vi "Download_Manager.vi"(7 "Downloader Exit":refnum<user-event>, 11 "manager_daemon":refnum<class "manager_daemon.lvclass">) -> ()   [LabVIEW 2024, in "Download_Manager.lvlib"]
uses:
  Download_Manager.lvlib
  comic_manager/manager_daemon/manager_daemon.lvclass
  typedefs/job--cluster.ctl
  typedefs/job_type--enum.ctl
  <vilib>/addons/_JKI.lib/REST Client/classes/REST Client/REST Client.lvclass
  comic_manager/manager_daemon/manager_daemon.lvclass/manager_daemon.ctl
  <vilib>/addons/_JKI Toolkits/State Machine/_JKI_lib_State_Machine.llb/Select State(s)_err__jki_lib_state_machine.vi
  <vilib>/Utility/error.llb/Trim Whitespace One-Sided.vi
  CV_RESTful_Library/CV_RESTful_Lib.lvlib
  <userlib>/_OpenG.lib/string/string.llb/openg_string.lvlib
  CV_Shared_Library/CV_Shared_Library.lvlib
panel:
  in  "queue publisher":bool
  in  "Publisher ID":i32=31
  in  "pause":bool
  in  "Volume URL":string
  in  "paste from clipboard":bool
  out "current queue size":i32
  out "Approx Completion":timestamp format="%<%x %X>T"
  out "Crawler Running":bool
  out "Timer":dbl
  in  "add url":bool
  in  "Rebuild Job List":bool=TRUE
  out "files updated":string[](array[string])
  in  "start crawler":bool
  out "status":string
  in  "Exit":bool
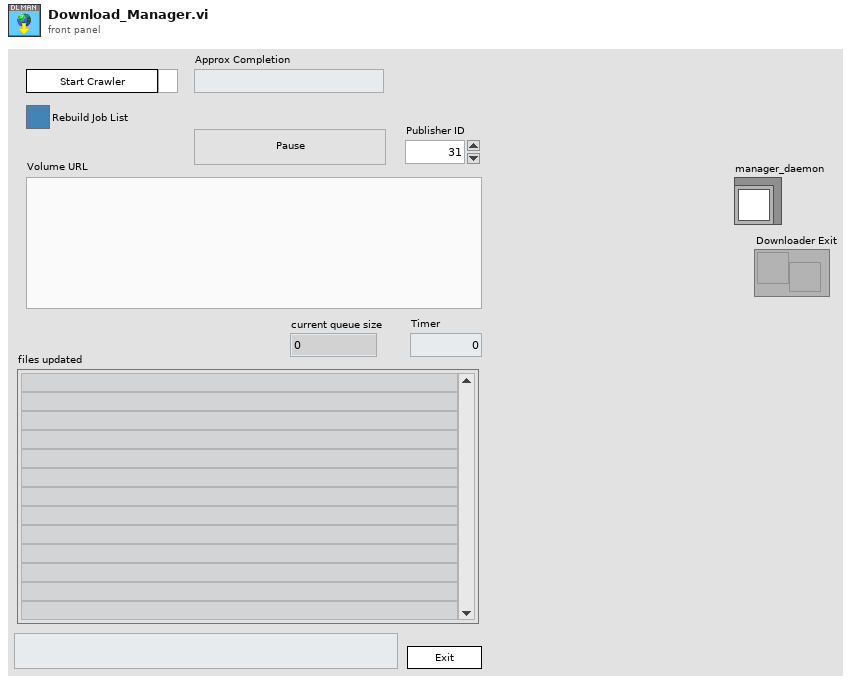
[diagram p1: front panel]
types:
  T1 = typedef "Download_Manager.lvlib/job_type--enum.ctl" = enum16{"check volume date", "check issues date", "download publisher", "download volume", "download isssue"}
  T2 = typedef "Download_Manager.lvlib/job--cluster.ctl" = cluster{"job type":T1, "job path":path, "id":i32, "url":string, "last updated":timestamp, "offset":i32, "original path":path}
  T3 = enum32{"Invalid", "Standard", "Closed", "Hidden", "Minimized", "Maximized"}
  T4 = enum32{"invalid app kind", "Development System", "Run Time System", "Student Edition", "Embedded LabVIEW", "Evaluation", "Custom"}
  T5 = cluster{"Core":cluster{"Current VI Reference":refnum<vi>, "Close Panel on Exit?":bool}, "TO":i32, "dl timer":u32, "cv_vol path":path, "cv_iss path":path, "cache folder":path, "REST Client":refnum<class "REST Client.lvclass">, "crawler active":bool, "job queue":refnum<queue>, "manager_daemon":refnum<class "manager_daemon.lvclass">, "status log ref":refnum<file>, "error log ref":refnum<file>, "ms delay":u32, "cv_pub path":path, "Downloader Exit":refnum<user-event>}
  T6 = cluster{"Current VI Reference":refnum<vi>, "Close Panel on Exit?":bool}
  T7 = typedef "CV_RESTful_Lib.lvlib/local_publisher--cluster.ctl" = cluster{"id":i32, "name":string, "sortable_name":string, "aliases":string[], "description":string, "deck":string, "site_detail_url":string, "date_last_updated":timestamp, "cv_id":string, "volume_ids":i32[]}
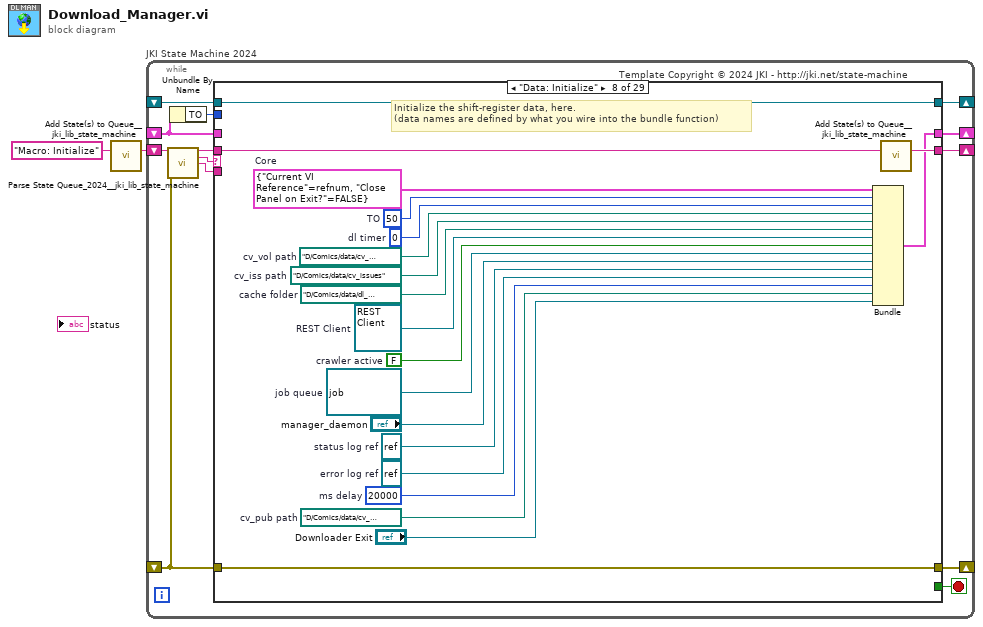
[diagram p0: block diagram]
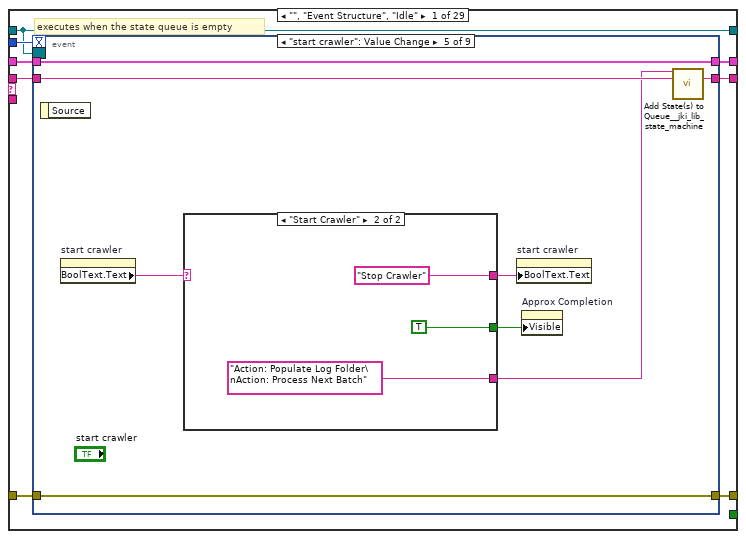
[diagram p2: hidden frame]
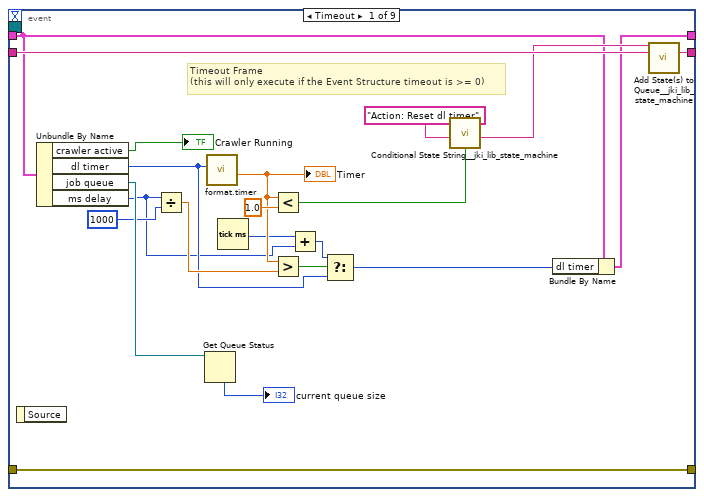
[diagram p3: hidden frame]
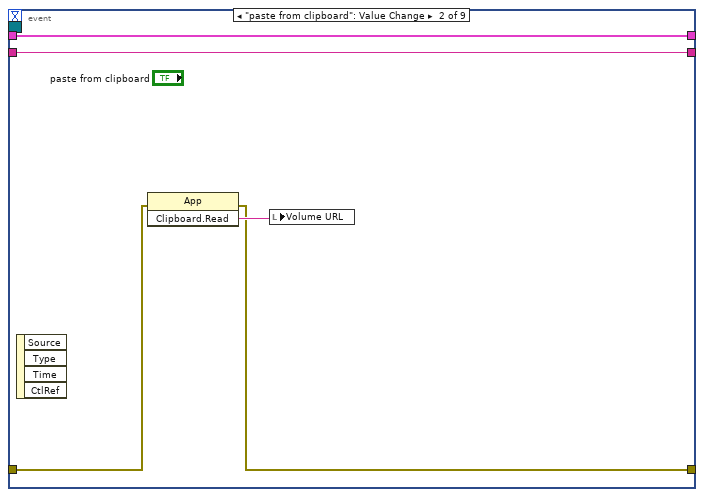
[diagram p4: hidden frame]
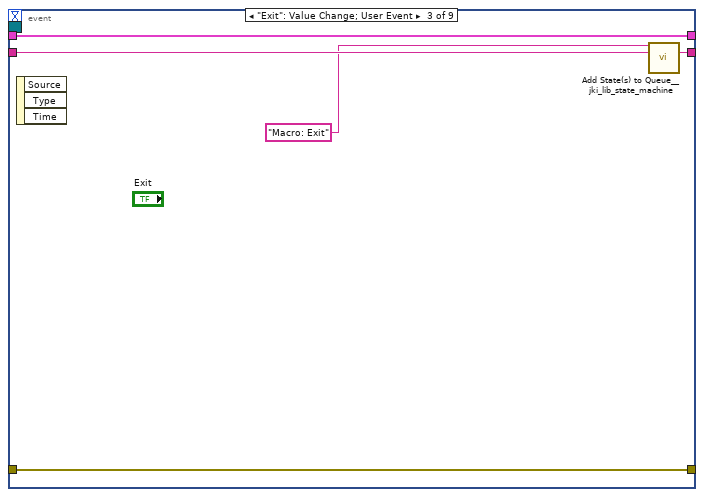
[diagram p5: hidden frame]
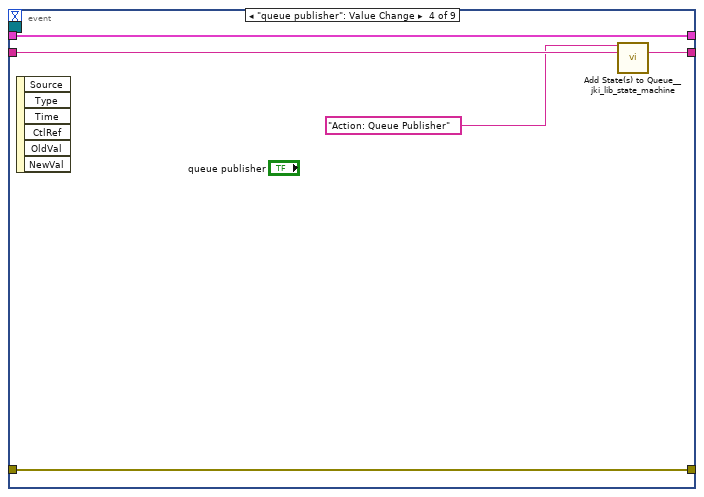
[diagram p6: hidden frame]
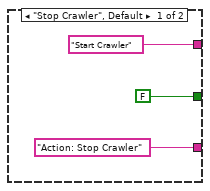
[diagram p7: hidden frame]
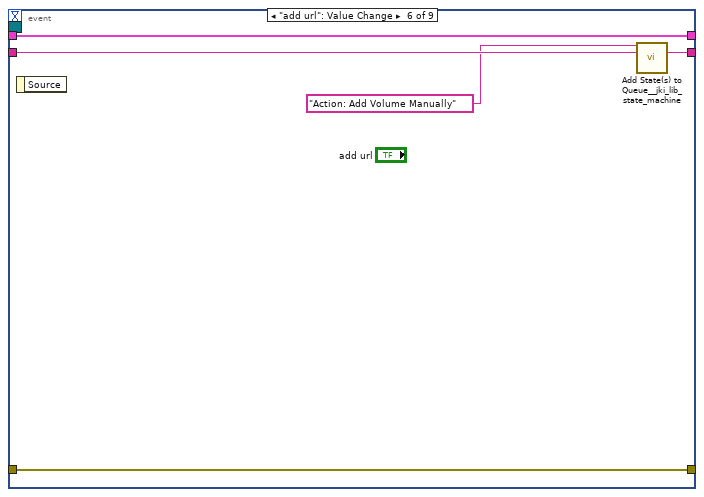
[diagram p8: hidden frame]
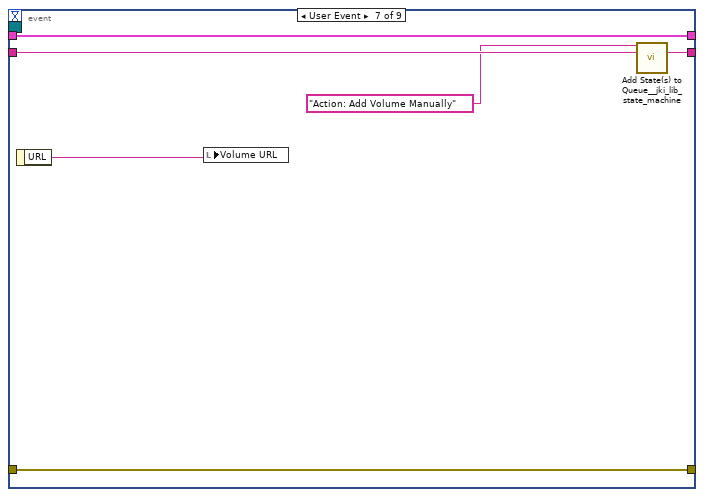
[diagram p9: hidden frame]
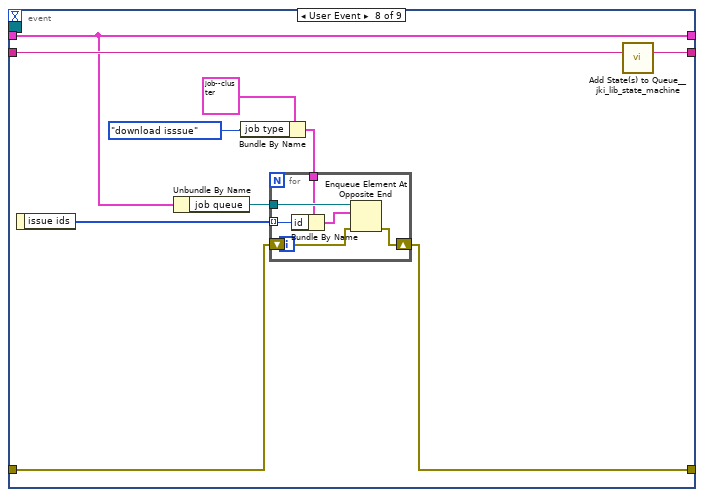
[diagram p10: hidden frame]
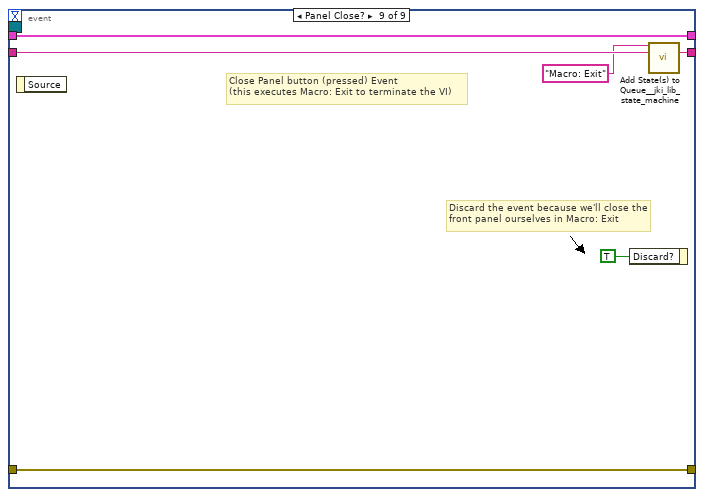
[diagram p11: hidden frame]
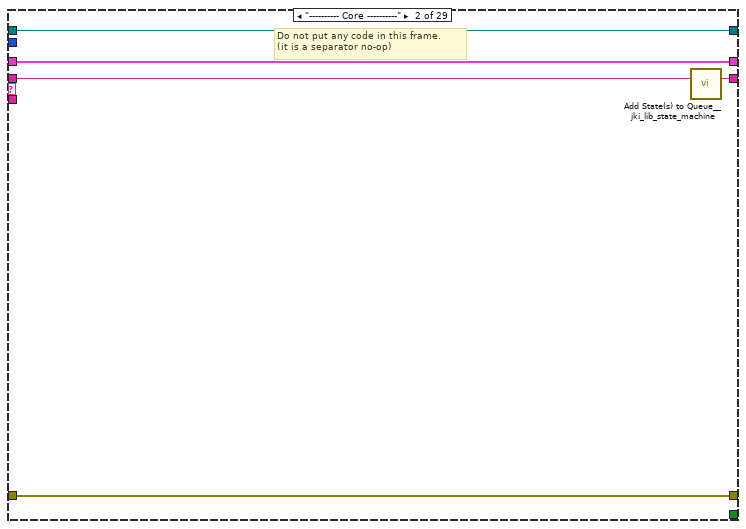
[diagram p12: hidden frame]
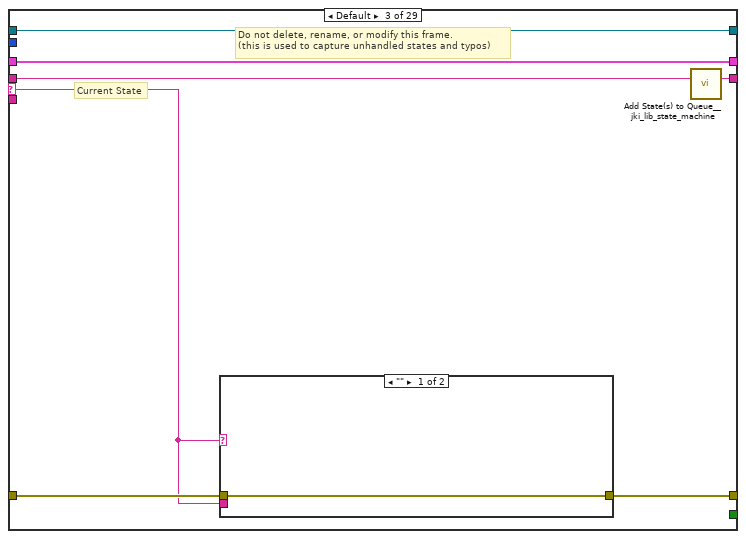
[diagram p13: hidden frame]
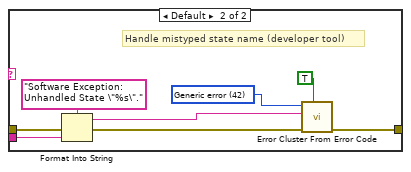
[diagram p14: hidden frame]
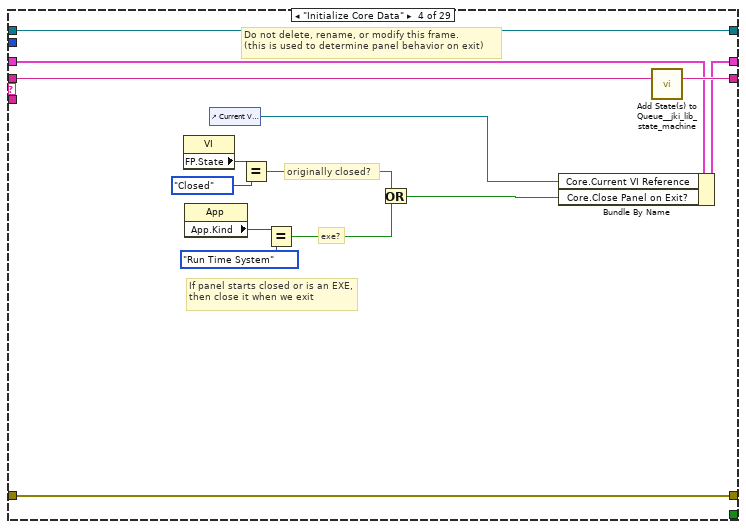
[diagram p15: hidden frame]
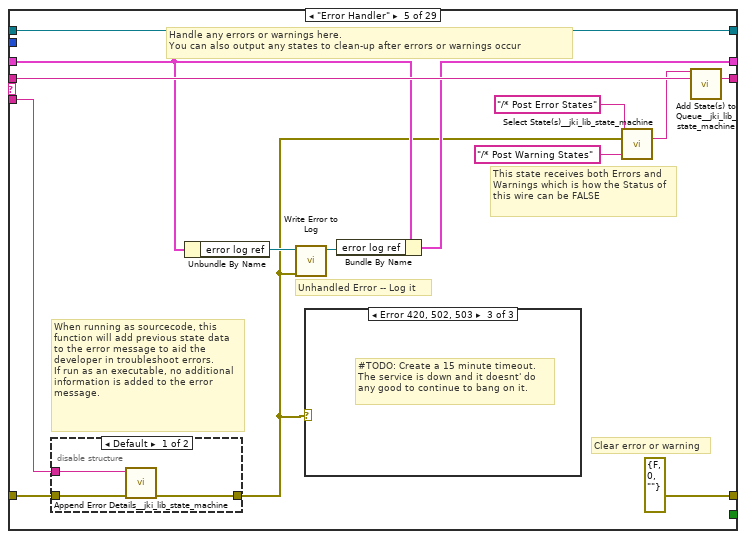
[diagram p16: hidden frame]
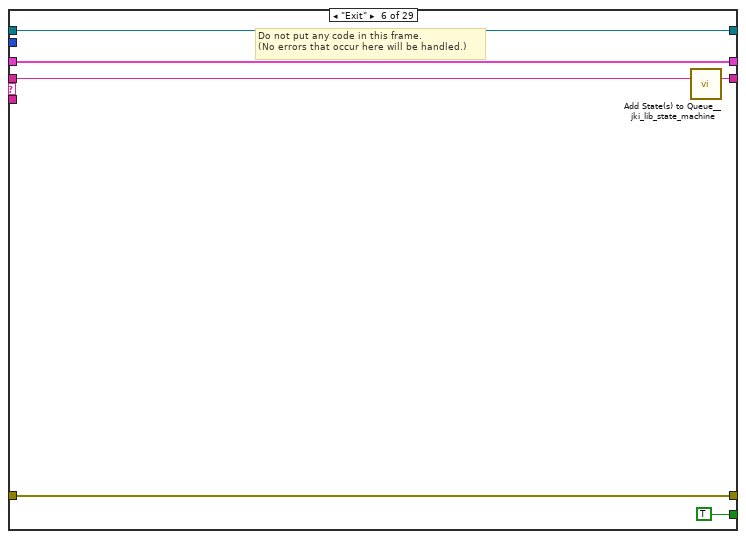
[diagram p20: hidden frame]
diagram:
  n1 = call <vilib>:"Add State(s) to Queue__jki_lib_state_machine.vi"("State(s) in (\"\")"="Macro: Initialize") -> ("States Out"=w2:string)  [unwired: 14 in]
  n2 = while "JKI State Machine 2024" {
    shift-right: [w8] -> _
    shift-left: _ -> [w5]
    shift-right: [w11] -> _
    shift-left: _ -> [w7]
    shift-right: [w10] -> _
    shift-left: w2 -> [w12]
    shift-right: [w4] -> _
    shift-left: _ -> [w3]
    stop <- w9 stop-if-true
    # "Template Copyright © 2024 JKI - http://jki.net/state-machine"
    n3 = call <vilib>:"Parse State Queue_2024__jki_lib_state_machine.vi"("State Queue"=w12, "Error In (no error)"=w7) -> ("Remaining States"=w14:string, "Current State"=w15:string, "Arguments"=w13:string)  [unwired: 11 in]
    n4 = Unbundle By Name(w5) -> ("TO"=w6:i32)
    n5 = case shown="\"Data: Initialize\"" w15 {
      selector: w15 -> [_ _ w113 _ _ _ _ _ _ _ _ _ _ _ _ _ _ _ _ _ _ _ _ _ _ _ _ _ _]
      tunnel: w14 -> [w23 w111 w116 w141 w155 w165 w170 w190 w202 w222 w227 w237 w243 w248 w257 w264 w271 w283 w353 w359 w369 w374 w394 w435 w464 w481 w499 w532 w548]
      tunnel: w13 -> [_ _ _ _ w151 _ _ _ _ _ _ _ _ _ _ _ w266 w277 _ _ _ _ _ _ _ _ _ _ _]
      tunnel: w5 -> [w21 w108 w114 w134 w144 w163 w167 _ w200 w218 w224 w233 w241 w245 w255 w262 w269 w279 w350 w356 w367 w371 w391 w431 w457 w474 w492 w528 w537]
      tunnel: [w20 w109 w118 w138 errorcluster {"status"=FALSE, "code"=0, "source"=""} ("error out") w162 w168 w187 w192 w219 w225 w234 w238 w246 w254 w261 w267 w280 w351 w357 w364 w372 w375 w421 w458 w476 w494 w516 w539] -> w11
      tunnel: w7 -> [w17 w109 w117 w138 w152 w162 w168 w187 w195 w206 w225 w235 w239 w246 w254 w261 w268 w281 w351 w357 w364 w372 w385 w416 w460 w478 w495 w530 w543]
      tunnel: [w22 w110 w115 w140 w154 w164 w169 w189 w201 w221 w226 w236 w242 w247 w256 w263 w270 w282 w352 w358 w368 w373 w393 w434 w463 w480 w498 w531 w547] -> w10
      tunnel: [_ _ _ _ _ TRUE _ _ _ _ _ _ _ _ _ _ _ _ _ _ _ _ _ _ _ _ _ _ _] -> w9
      tunnel: [w19 w108 w114 w139 w145 w163 w167 w188 w199 w218 w224 w233 w241 w245 w255 w262 w269 w279 w350 w356 w367 w371 w391 w424 w457 w474 w493 w527 w536] -> w8
      tunnel: w6 -> [w18 _ _ _ _ _ _ _ _ _ _ _ _ _ _ _ _ _ _ _ _ _ _ _ _ _ _ _ _]
      tunnel: [w16 w107 w112 w128 w143 w160 w166 w173 w191 w209 w223 w228 w240 w244 w250 w258 w265 w276 w349 w354 w360 w370 w392 w418 w456 w471 w490 w511 w533] -> w4
      tunnel: w3 -> [w16 w107 w112 w128 w143 w160 w166 w173 w191 w209 w223 _ w240 w244 w250 w258 w265 w276 w349 w354 w360 w370 w392 w418 w456 w471 w490 w511 w533]
      frame "", "Event Structure", "Idle" {
        # "executes when the state queue is empty"
        n6 = event shown="[4] \"start crawler\": Value Change" {
          selector: w16 -> [_ _ _ _ _ _ _ _ _]
          dyn-events: _ -> [_ _ _ _ _ _ _ _ _]
          timeout: w18 -> [_ _ _ _ _ _ _ _ _]
          tunnel: w23 -> [w44 w48 w54 w58 w67 w77 w83 w94 w106]
          tunnel: [w43 w48 w53 w57 w66 w76 w82 w93 w105] -> w22
          tunnel: w21 -> [w26 w49 w51 w59 w60 w78 w84 w92 w103]
          tunnel: [w42 w46 w52 w55 w65 w74 w80 w85 w104] -> w20
          tunnel: w17 -> [w42 w45 w52 w55 w65 w74 w80 w86 w104]
          tunnel: [w24 w49 w51 w59 w60 w78 w84 w92 w103] -> w19
          event Timeout {
            # "Timeout Frame\n(this will only execute if the Event Structure timeout is >= 0)"
            n7 = event-data() -> ()  [unwired: 1 in, 1 out]
            n8 = Unbundle By Name(w26) -> ("crawler active"=→"Crawler Running":bool, "dl timer"=w30:u32, "job queue"=w36:refnum<queue>, "ms delay"=w28:u32)
            n9 = Divide(x=w28, y=u32 1000) -> (x/y=w32:dbl)
            n10 = Get Queue Status(queue=w36) -> (# elements in queue=→"current queue size":i32)  [unwired: 2 in, 7 out]
            n11 = call "format.timer.vi"("dl timer"=w30) -> ("seconds"=w34:dbl)  [unwired: 10 in]
            "Timer" <- w34
            n12 = Tick Count (ms)() -> (millisecond timer value=w29:u32)
            n13 = Less?(x=w34, y=1.0) -> (x < y?=w40:bool)
            n14 = Greater?(x=w34, y=w32) -> (0:w31:bool)
            n15 = Add(x=w29, y=w28) -> (x+y=w27:u32)
            n16 = Select(t=w27, s=w31, f=w30) -> (s? t:f=w25:u32)
            n17 = call <vilib>:"Conditional State String__jki_lib_state_machine.vi"("Do State(s)?"=w40, "State"="Action: Reset dl timer") -> ("State Out"=w39:string)  [unwired: 7 in]
            n18 = Bundle By Name(cluster=w26, "dl timer"=w25) -> (w24:T5)
            n19 = call <vilib>:"Add State(s) to Queue__jki_lib_state_machine.vi"("State(s) in Front (\"\")"=w39, "State(s) in (\"\")"=w44) -> ("States Out"=w43:string)  [unwired: 13 in]
          }
          event "paste from clipboard": Value Change {
            n20 = event-data() -> ()  [unwired: 1 in, 4 out]
            n21 = invoke class="App" method="Clipboard.Read"(error in=w45) -> (error out=w46:errorcluster, "Read Clipbrd"=w47:string)  [unwired: 2 in, 1 out]
            n22 = local write "Volume URL"(w47) -> ()
          }
          event "Exit": Value Change; User Event {
            n23 = event-data() -> ()  [unwired: 1 in, 3 out]
            n24 = call <vilib>:"Add State(s) to Queue__jki_lib_state_machine.vi"("State(s) in Front (\"\")"="Macro: Exit", "State(s) in (\"\")"=w54) -> ("States Out"=w53:string)  [unwired: 13 in]
          }
          event "queue publisher": Value Change {
            n25 = event-data() -> ()  [unwired: 1 in, 6 out]
            n26 = call <vilib>:"Add State(s) to Queue__jki_lib_state_machine.vi"("State(s) in Front (\"\")"="Action: Queue Publisher" ("State(s) in Front (\"\")"), "State(s) in (\"\")"=w58) -> ("States Out"=w57:string)  [unwired: 13 in]
          }
          event "start crawler": Value Change {
            n27 = event-data() -> ()  [unwired: 1 in, 1 out]
            n28 = property on="start crawler" class="Bool"() -> ("BoolText.Text"=w63:string)  [unwired: 2 in, 2 out]
            n29 = case shown="\"Start Crawler\"" w63 {
              tunnel: ["Action: Stop Crawler" "Action: Populate Log Folder\nAction: Process Next Batch"] -> w64
              tunnel: [FALSE ("Visible") TRUE ("Visible")] -> w62
              tunnel: ["Start Crawler" ("Boolean Text.Text") "Stop Crawler" ("Boolean Text.Text")] -> w61
              frame "Stop Crawler", Default {
              }
              frame "Start Crawler" {
              }
            }
            n30 = property on="start crawler" class="Bool"("BoolText.Text"=w61) -> ()  [unwired: 2 in, 2 out]
            n31 = property on="Approx Completion" class="AbsTime (strict)"("Visible"=w62) -> ()  [unwired: 2 in, 2 out]
            n32 = call <vilib>:"Add State(s) to Queue__jki_lib_state_machine.vi"("State(s) in Front (\"\")"=w64, "State(s) in (\"\")"=w67) -> ("States Out"=w66:string)  [unwired: 13 in]
          }
          event "add url": Value Change {
            n33 = event-data() -> ()  [unwired: 1 in, 1 out]
            n34 = call <vilib>:"Add State(s) to Queue__jki_lib_state_machine.vi"("State(s) in Front (\"\")"="Action: Add Volume Manually" ("State"), "State(s) in (\"\")"=w77) -> ("States Out"=w76:string)  [unwired: 13 in]
          }
          event User Event {
            n35 = event-data() -> ("URL"=w79:string)  [unwired: 1 in]
            n36 = local write "Volume URL"(w79) -> ()
            n37 = call <vilib>:"Add State(s) to Queue__jki_lib_state_machine.vi"("State(s) in Front (\"\")"="Action: Add Volume Manually" ("State"), "State(s) in (\"\")"=w83) -> ("States Out"=w82:string)  [unwired: 13 in]
          }
          event User Event {
            n38 = event-data() -> ("issue ids"=w91:i32[])  [unwired: 1 in]
            n39 = Unbundle By Name(w92) -> ("job queue"=w88:refnum<queue>)
            n40 = Bundle By Name(cluster=T2 {"job type"=enum."check volume date", "job path"=path "", "id"=0, "url"="", "last updated"=timestamp(0 s since 1904-01-01), "offset"=0, "original path"=path ""} ("element"), "job type"=job_type--enum."download isssue") -> (w87:T2)
            n41 = for {
              tunnel: w91 -> [w98] mode=indexing
              tunnel: w88 -> [w100]
              tunnel: w87 -> [w99]
              shift-right: [w95] -> w85
              shift-left: w86 -> [w96]
              n42 = Bundle By Name(cluster=w99, "id"=w98) -> (w97:T2)
              n43 = Enqueue Element At Opposite End(queue=w100, element=w97, error in (no error)=w96) -> (error out=w95:errorcluster)  [unwired: 1 in, 2 out]
            }
            n44 = call <vilib>:"Add State(s) to Queue__jki_lib_state_machine.vi"("State(s) in (\"\")"=w94) -> ("States Out"=w93:string)  [unwired: 14 in]
          }
          event Panel Close? {
            # "Discard the event because we'll close the front panel ourselves in Macro: Exit"
            # "Close Panel button (pressed) Event\n(this executes Macro: Exit to terminate the VI)"
            n45 = event-data() -> ()  [unwired: 1 in, 1 out]
            n46 = event-data("Discard?"=TRUE) -> ()  [unwired: 1 in, 1 out]
            n47 = call <vilib>:"Add State(s) to Queue__jki_lib_state_machine.vi"("State(s) in Front (\"\")"="Macro: Exit", "State(s) in (\"\")"=w106) -> ("States Out"=w105:string)  [unwired: 13 in]
          }
        }
      }
      frame "---------- Core ----------" {
        # "Do not put any code in this frame.\n(it is a separator no-op)"
        n48 = call <vilib>:"Add State(s) to Queue__jki_lib_state_machine.vi"("State(s) in (\"\")"=w111) -> ("States Out"=w110:string)  [unwired: 14 in]
      }
      frame Default {
        # "Current State"
        # "Do not delete, rename, or modify this frame.\n(this is used to capture unhandled states and typos)"
        n49 = case shown="\"\"" w113 {
          tunnel: [w119 w123] -> w118
          tunnel: w117 -> [w119 w122]
          tunnel: w113 -> [_ w120]
          frame "" {
          }
          frame Default {
            w126 = 42 items=["No error", "Argument error", "Memory is full", "Out of zone", "End of file", "File already open", "Generic file I/O error", "File not found", "File permission error", "Disk is full", "Duplicate path", "Too many files open", "System feature not enabled", "Resource file not found", "Cannot add resource", "Resource not found", "Image not found", "Image memory error", "Pen does not exist", "Config type invalid", "Config token not found", "Config parse error", "Config memory error", "Bad external code format", "Bad external code offset", "External code not present", "Null window", "Destroy window error", "Null menu", "Print aborted", "Bad print record", "Print driver error", "Windows error during printing", "Memory error during printing", "Print dialog error", "Generic print error", "Invalid device refnum", "Device not found", "Device parameter error", "Device unit error", "Cannot open device", "Device call aborted", "Generic error", "Cancelled by user", "Object ID too low", "Object ID too high", "Object not in heap", "Unknown heap", "Unknown object (invalid DefProc)", "Unknown object (DefProc not in table)", "Message out of range", "Invalid (null) method", "Unknown message", "Manager call not supported", "Bad address", "Network operation in progress", "Network operation timed out", "Connection is busy", "Network attribute not supported", "Network error", "Address in use", "System out of memory", "Connection aborted", "Connection refused", "Not connected", "Already connected", "Connection closed", "Initialization error (interapplication manager)", "Bad occurrence", "Wait on unbound occurrence handler", "Occurrence queue overflow", "Datalog type conflict", "Unused", "Unrecognized type (interapplication manager)", "Memory corrupt", "Failed to make temporary DLL", "Old CIN version", "Drag socket not found", "Failed to load drop-object", "Failed to register OLE object", "Failed to release OLE object", "Format specifier type mismatch", "Unknown format specifier", "Too few format specifiers", "Too many format specifiers", "Scan failed", "Newer CIN version", "Error converting to variant", "Runtime menu error", "Password tampered", "Variant attribute not found", "Incompatible variant data type", "Event data is not available", "Event Store is not present", "Occurrence is not found", "Event Queue is not created", "Event info is not available", "Refnum passed is NULL", "Error retrieving Class GUID", "Error retrieving CoClass GUID", "Error retrieving TypeLib GUID.", "Bad built application magic bytes.", "Specific driver is different from the specific driver associated with the Logical Name.", "There is no session opened to the class driver.", "Max Error", "MAX - Error with config objects", "MAX - Error loading configuration", "MAX - Group not supported"]
            # "Handle mistyped state name (developer tool)"
            n50 = Format Into String(format string="Software Exception: Unhandled State \"%s\"." ("message"), error in=w122, w120) -> (resulting string=w125:string, error out=w124:errorcluster)  [unwired: 1 in]
            n51 = call <vilib>:"Error Cluster From Error Code.vi"("show call chain? (False)"=TRUE, "error in (no error)"=w124, "error message (\"\")"=w125, "error code (0)"=w126) -> ("error out"=w123:errorcluster)  [unwired: 5 in]
          }
        }
        n52 = call <vilib>:"Add State(s) to Queue__jki_lib_state_machine.vi"("State(s) in (\"\")"=w116) -> ("States Out"=w115:string)  [unwired: 14 in]
      }
      frame "Initialize Core Data" {
        # "Do not delete, rename, or modify this frame.\n(this is used to determine panel behavior on exit)"
        # "originally closed?"
        # "exe?"
        # "If panel starts closed or is an EXE, then close it when we exit"
        n53 = property class="VI"() -> ("FP.State"=w131:T3)  [unwired: 2 in, 2 out]
        n54 = property class="App"() -> ("App.Kind"=w137:T4)  [unwired: 2 in, 2 out]
        n55 = control-ref of="Current VI Reference"() -> (w132:refnum<vi>)
        n56 = Equal?(x=w131, y=T3."Closed" ("Front Panel Window:State")) -> (x = y?=w129:bool)
        n57 = Equal?(x=w137, y=T4."Run Time System" ("Application:Kind")) -> (x = y?=w135:bool)
        n58 = Or(x=w129, y=w135) -> (x .or. y?=w133:bool)
        n59 = Bundle By Name(cluster=w134, "Core.Current VI Reference"=w132, "Core.Close Panel on Exit?"=w133) -> (w139:T5)
        n60 = call <vilib>:"Add State(s) to Queue__jki_lib_state_machine.vi"("State(s) in (\"\")"=w141) -> ("States Out"=w140:string)  [unwired: 14 in]
      }
      frame "Error Handler" {
        # "When running as sourcecode, this function will add previous state data to the error message to aid the developer in troubleshoot errors.\nIf run as an executable, no additional information is added to the error message."
        # "This state receives both Errors and Warnings which is how the Status of this wire can be FALSE"
        # "Unhandled Error -- Log it"
        # "Handle any errors or warnings here.\nYou can also output any states to clean-up after errors or warnings occur"
        # "Clear error or warning"
        n61 = disable-structure shown="Default" {
          disable-tunnel: w152 -> [w158 w159]
          disable-tunnel: w151 -> [w157 _]
          disable-tunnel: [w156 w159] -> w142
          frame condition #0 (active) {
            n62 = call <vilib>:"Append Error Details__jki_lib_state_machine.vi"("error in (no error)"=w158, "Previous State and Argument(s)"=w157) -> ("error out"=w156:errorcluster)  [unwired: 9 in]
          }
          frame condition #1 {
          }
        }
        n63 = Unbundle By Name(w144) -> ("error log ref"=w147:refnum<file>)
        n64 = call "Write Error to Log.vi"("error in (no error)"=w142, "file reference in"=w147) -> ("file reference out"=w146:refnum<file>)  [unwired: 8 in, 1 out]
        n65 = case shown="Error 420, 502, 503" w142 {
          frame No Error {
          }
          frame Default {
          }
          frame Error {
            # "#TODO: Create a 15 minute timeout.\nThe service is down and it doesnt' do\nany good to continue to bang on it."
          }
        }
        n66 = Bundle By Name(cluster=w144, "error log ref"=w146) -> (w145:T5)
        n67 = call-poly <vilib>:"Select State(s)__jki_lib_state_machine.vi"("State(s) if True (\"\")"="/* Post Error States", "Select"=w142, "State(s) if False (\"\")"="/* Post Warning States") -> ("States Out"=w149:string)  [unwired: 12 in]
        n68 = call <vilib>:"Add State(s) to Queue__jki_lib_state_machine.vi"("State(s) in Front (\"\")"=w149, "State(s) in (\"\")"=w155) -> ("States Out"=w154:string)  [unwired: 13 in]
      }
      frame "Exit" {
        # "Do not put any code in this frame.\n(No errors that occur here will be handled.)"
        n69 = call <vilib>:"Add State(s) to Queue__jki_lib_state_machine.vi"("State(s) in (\"\")"=w165) -> ("States Out"=w164:string)  [unwired: 14 in]
      }
      frame "---------- Data ----------" {
        # "Do not put any code in this frame.\n(It is a separator no-op. You can make a copy of this frame to create a new Data frame)"
        n70 = call <vilib>:"Add State(s) to Queue__jki_lib_state_machine.vi"("State(s) in (\"\")"=w170) -> ("States Out"=w169:string)  [unwired: 14 in]
      }
      frame "Data: Initialize" {
        w172 = path "D:/Comics/data/cv_publishers"  # cv_pub path
        w174 = u32 20000  # ms delay
        w175 = refnum<file> refnum  # error log ref
        w176 = refnum<file> refnum  # status log ref
        w178 = refnum<queue> refnum  # job queue
        w179 = FALSE  # crawler active
        w180 = refnum<class "REST Client.lvclass"> refnum  # REST Client
        w181 = path "D:/Comics/data/dl_manager"  # cache folder
        w182 = path "D:/Comics/data/cv_issues"  # cv_iss path
        w183 = path "D:/Comics/data/cv_volumes"  # cv_vol path
        w184 = u32 0  # dl timer
        w185 = 50  # TO
        w186 = T6 {"Current VI Reference"=refnum, "Close Panel on Exit?"=FALSE}  # Core
        # "Initialize the shift-register data, here.\n(data names are defined by what you wire into the bundle function)"
        n71 = Bundle("Core"=w186, "TO"=w185, "dl timer"=w184, "cv_vol path"=w183, "cv_iss path"=w182, "cache folder"=w181, "REST Client"=w180, "crawler active"=w179, "job queue"=w178, "manager_daemon"="manager_daemon", "status log ref"=w176, "error log ref"=w175, "ms delay"=w174, "cv_pub path"=w172, "Downloader Exit"="Downloader Exit") -> (w188:T5)  [unwired: 1 in]
        n72 = call <vilib>:"Add State(s) to Queue__jki_lib_state_machine.vi"("State(s) in (\"\")"=w190) -> ("States Out"=w189:string)  [unwired: 14 in]
      }
      frame "Data: Init Objects" {
        n73 = Obtain Queue(element data type=T2 {"job type"=enum."check volume date", "job path"=path "", "id"=0, "url"="", "last updated"=timestamp(0 s since 1904-01-01), "offset"=0, "original path"=path ""} ("job")) -> (queue out=w196:refnum<queue>, error out=w194:errorcluster)  [unwired: 4 in, 1 out]
        n74 = call "Open_RESTful_connection.vi"("error in (no error)"=w195) -> ("error out"=w193:errorcluster, "REST Client out"=w198:refnum<class "REST Client.lvclass">)  [unwired: 9 in]
        n75 = Merge Errors(w193, w194) -> (w192:errorcluster)
        n76 = Bundle By Name(cluster=w200, "REST Client"=w198, "job queue"=w196) -> (w199:T5)
        n77 = call <vilib>:"Add State(s) to Queue__jki_lib_state_machine.vi"("State(s) in (\"\")"=w202) -> ("States Out"=w201:string)  [unwired: 14 in]
      }
      frame "Data: Cleanup" {
        # "Cleanup any data and references, here.\n(this is called automatically, by the Macro: Exit)"
        n78 = Unbundle By Name(w218) -> ("Core.Current VI Reference"=w220:refnum<vi>, "REST Client"=w217:refnum<class "REST Client.lvclass">, "job queue"=w215:refnum<queue>, "status log ref"=w210:refnum<file>, "error log ref"=w213:refnum<file>, "Downloader Exit"=w208:refnum<user-event>)
        n79 = Generate User Event(user event=w208, event data cluster=TRUE ("event data"), error in=w206) -> (error out=w205:errorcluster)  [unwired: 1 in, 1 out]
        n80 = call <vilib>:"Clear Errors.vi"("error in (no error)"=w205, "specific error code to clear (0: all)"=1) -> ("error out"=w203:errorcluster)  [unwired: 4 in, 1 out]
        n81 = Close File(refnum=w213, error in=w203) -> (error out=w212:errorcluster)  [unwired: 1 out]
        n82 = Close File(refnum=w210, error in=w212) -> (error out=w211:errorcluster)  [unwired: 1 out]
        n83 = Release Queue(queue=w215, error in (no error)=w211) -> (error out=w214:errorcluster)  [unwired: 1 in, 2 out]
        n84 = call-dynamic "Destroy REST Client.vi"("error in (no error)"=w214, "REST Client in"=w217) -> ("error out"=w216:errorcluster)  [unwired: 9 in]
        n85 = Close Reference(reference=w220, error in (no error)=w216) -> (error out=w219:errorcluster)
        n86 = call <vilib>:"Add State(s) to Queue__jki_lib_state_machine.vi"("State(s) in (\"\")"=w222) -> ("States Out"=w221:string)  [unwired: 14 in]
      }
      frame "---------- Events ----------" {
        # "Do not put any code in this frame.\n(It is a separator no-op. You can make a copy of this frame to create a new UI frame)"
        n87 = call <vilib>:"Add State(s) to Queue__jki_lib_state_machine.vi"("State(s) in (\"\")"=w227) -> ("States Out"=w226:string)  [unwired: 14 in]
      }
      frame "Events: Register" {
        # "Do not put any code in this frame.\n(It is a separator no-op. You can make a copy of this frame to create a new UI frame)"
        n88 = Unbundle By Name(w233) -> ("manager_daemon"=w232:refnum<class "manager_daemon.lvclass">, "Downloader Exit"=w229:refnum<user-event>)
        n89 = call "DL_events.get.vi"("manager_daemon in"=w232) -> ("download issues event"=w230:refnum<user-event>, "volume url event"=w231:refnum<user-event>)  [unwired: 8 in, 1 out]
        n90 = register-events(error in=w235, w231, w230, w229) -> (reference out=w228:refnum<event-registration>, error out=w234:errorcluster)  [unwired: 1 in]
        n91 = call <vilib>:"Add State(s) to Queue__jki_lib_state_machine.vi"("State(s) in (\"\")"=w237) -> ("States Out"=w236:string)  [unwired: 14 in]
      }
      frame "Events: Unregister" {
        # "Do not put any code in this frame.\n(It is a separator no-op. You can make a copy of this frame to create a new UI frame)"
        n92 = Unregister For Events(event registration refnum=w240, error in=w239) -> (error out=w238:errorcluster)
        n93 = call <vilib>:"Add State(s) to Queue__jki_lib_state_machine.vi"("State(s) in (\"\")"=w243) -> ("States Out"=w242:string)  [unwired: 14 in]
      }
      frame "---------- UI ----------" {
        # "Do not put any code in this frame.\n(It is a separator no-op. You can make a copy of this frame to create a new UI frame)"
        n94 = call <vilib>:"Add State(s) to Queue__jki_lib_state_machine.vi"("State(s) in (\"\")"=w248) -> ("States Out"=w247:string)  [unwired: 14 in]
      }
      frame "UI: Initialize" {
        w249 = FALSE ("Visible")
        # "Initialize the User Interface, here.\n(this is called automatically, by the Macro: Initialize)"
        n95 = property on="start crawler" class="Bool"("BoolText.Text"="Start Crawler" ("Boolean Text.Text")) -> ()  [unwired: 2 in, 2 out]
        n96 = local write "Crawler Running"(FALSE ("Crawler Running")) -> ()
        n97 = property on="Approx Completion" class="AbsTime (strict)"("Visible"=w249) -> ()  [unwired: 2 in, 2 out]
        n98 = property on="manager_daemon" class="LVClassControl (strict)"("Visible"=w249) -> ()  [unwired: 2 in, 2 out]
        n99 = local write "files updated"(string[] []) -> ()
        n100 = call <vilib>:"Add State(s) to Queue__jki_lib_state_machine.vi"("State(s) in (\"\")"=w257) -> ("States Out"=w256:string)  [unwired: 14 in]
      }
      frame "UI: Uninitialize" {
        # "Cleanup the User Interface, here.\n(this is called automatically, by the Macro: Exit)"
        n101 = property on="Approx Completion" class="AbsTime (strict)"("Visible"=TRUE) -> ()  [unwired: 2 in, 2 out]
        n102 = property on="manager_daemon" class="LVClassControl (strict)"("Visible"=TRUE) -> ()  [unwired: 2 in, 2 out]
        n103 = call <vilib>:"Add State(s) to Queue__jki_lib_state_machine.vi"("State(s) in (\"\")"=w264) -> ("States Out"=w263:string)  [unwired: 14 in]
      }
      frame "UI: Cursor Set" {
        # "Argument"
        # "Set and Unset Cursor Busy.\n(Usage: \"UI: Cursor Set >> Busy|Idle\")"
        n104 = case shown="\"Idle\", Default" w266 {
          tunnel: w268 -> [w273 w275]
          tunnel: [w272 w274] -> w267
          frame "Idle", Default {
            n105 = call <vilib>:"Unset Busy.vi"("error in (no error)"=w273) -> ("error out"=w272:errorcluster)  [unwired: 10 in]
          }
          frame "Busy" {
            n106 = call <vilib>:"Set Busy.vi"("error in (no error)"=w275) -> ("error out"=w274:errorcluster)  [unwired: 9 in, 1 out]
          }
        }
        n107 = call <vilib>:"Add State(s) to Queue__jki_lib_state_machine.vi"("State(s) in (\"\")"=w271) -> ("States Out"=w270:string)  [unwired: 14 in]
      }
      frame "UI: Front Panel State" {
        # "Argument"
        # "Set Front Panel Open or Closed\n(Usage: \"UI: Front Panel State >> Open|Close\")"
        n108 = Unbundle By Name(w279) -> ("Core.Current VI Reference"=w278:refnum<vi>)
        n109 = case shown="\"Open\", \"Standard\", Default" w277 {
          tunnel: w281 -> [w289 w304 w315 w328 w341]
          tunnel: [w291 w305 w317 w330 w343] -> w280
          tunnel: w278 -> [w290 w302 w316 w329 w342]
          frame "Open", "Standard", Default {
            w284 = T3."Standard" ("State")
            n110 = property class="VI"(reference=w290, error in=w289) -> (reference out=w287:refnum<vi>, error out=w288:errorcluster, "FP.State"=w286:T3)
            n111 = Not Equal?(x=w286, y=w284) -> (x != y?=w285:bool)
            n112 = case shown="True" w285 {
              tunnel: [w295 w297] -> w291
              tunnel: w288 -> [w294 w297]
              tunnel: w287 -> [w293 _]
              tunnel: w284 -> [w292 _]
              frame True {
                n113 = invoke class="VI" method="FP.Open"(reference=w293, error in=w294, "Activate"=TRUE, "State"=w292) -> (error out=w295:errorcluster)  [unwired: 1 in, 4 out]
              }
              frame False {
              }
            }
          }
          frame "Close", "Closed" {
            n114 = property class="VI"(reference=w302, error in=w304) -> (reference out=w301:refnum<vi>, error out=w303:errorcluster, "FP.State"=w299:T3)
            n115 = Not Equal?(x=w299, y=T3."Closed" ("Front Panel Window:State")) -> (x != y?=w298:bool)
            n116 = case shown="True" w298 {
              tunnel: [w306 w309] -> w305
              tunnel: w303 -> [w306 w308]
              tunnel: w301 -> [_ w307]
              frame False {
              }
              frame True {
                n117 = invoke class="VI" method="FP.Close"(reference=w307, error in=w308) -> (error out=w309:errorcluster)  [unwired: 1 in, 2 out]
              }
            }
          }
          frame "Hidden", "Hide" {
            w310 = T3."Hidden" ("State")
            n118 = property class="VI"(reference=w316, error in=w315) -> (reference out=w313:refnum<vi>, error out=w314:errorcluster, "FP.State"=w312:T3)
            n119 = Not Equal?(x=w312, y=w310) -> (x != y?=w311:bool)
            n120 = case shown="True" w311 {
              tunnel: [w321 w322] -> w317
              tunnel: w314 -> [w320 w322]
              tunnel: w313 -> [w319 _]
              tunnel: w310 -> [w318 _]
              frame True {
                n121 = invoke class="VI" method="FP.Open"(reference=w319, error in=w320, "State"=w318) -> (error out=w321:errorcluster)  [unwired: 2 in, 4 out]
              }
              frame False {
              }
            }
          }
          frame "Minimize", "Minimized" {
            w323 = T3."Minimized" ("State")
            n122 = property class="VI"(reference=w329, error in=w328) -> (reference out=w326:refnum<vi>, error out=w327:errorcluster, "FP.State"=w325:T3)
            n123 = Not Equal?(x=w325, y=w323) -> (x != y?=w324:bool)
            n124 = case shown="True" w324 {
              tunnel: [w334 w335] -> w330
              tunnel: w327 -> [w333 w335]
              tunnel: w326 -> [w332 _]
              tunnel: w323 -> [w331 _]
              frame True {
                n125 = invoke class="VI" method="FP.Open"(reference=w332, error in=w333, "State"=w331) -> (error out=w334:errorcluster)  [unwired: 2 in, 4 out]
              }
              frame False {
              }
            }
          }
          frame "Maximize", "Maximized" {
            w336 = T3."Maximized" ("State")
            n126 = property class="VI"(reference=w342, error in=w341) -> (reference out=w339:refnum<vi>, error out=w340:errorcluster, "FP.State"=w338:T3)
            n127 = Not Equal?(x=w338, y=w336) -> (x != y?=w337:bool)
            n128 = case shown="True" w337 {
              tunnel: [w347 w348] -> w343
              tunnel: w340 -> [w346 w348]
              tunnel: w339 -> [w345 _]
              tunnel: w336 -> [w344 _]
              frame True {
                n129 = invoke class="VI" method="FP.Open"(reference=w345, error in=w346, "State"=w344) -> (error out=w347:errorcluster)  [unwired: 2 in, 4 out]
              }
              frame False {
              }
            }
          }
        }
        n130 = call <vilib>:"Add State(s) to Queue__jki_lib_state_machine.vi"("State(s) in (\"\")"=w283) -> ("States Out"=w282:string)  [unwired: 14 in]
      }
      frame "---------- Macro ----------" {
        # "Do not put any code in this frame.\n(It is a separator no-op. You can make a copy of this frame to create a new Macro frame)"
        n131 = call <vilib>:"Add State(s) to Queue__jki_lib_state_machine.vi"("State(s) in (\"\")"=w353) -> ("States Out"=w352:string)  [unwired: 14 in]
      }
      frame "Macro: Initialize" {
        # "Initialization Macro\n(This is called once, when the VI starts)"
        n132 = call <vilib>:"Add State(s) to Queue__jki_lib_state_machine.vi"("State(s) in Front (\"\")"="Data: Initialize\nData: Init Objects\nInitialize Core Data\nEvents: Register\nAction: Reset dl timer\nUI: Initialize\nUI: Front Panel State >> Open", "State(s) in (\"\")"=w359) -> ("States Out"=w358:string)  [unwired: 13 in]
      }
      frame "Macro: Exit" {
        # "Exit Macro\n(This is called once, when the VI exits)"
        n133 = Unbundle By Name(w367) -> ("Core.Close Panel on Exit?"=w362:bool)
        n134 = call <vilib>:"Conditional State String__jki_lib_state_machine.vi"("Do State(s)?"=w362, "State"="UI: Front Panel State >> Close") -> ("State Out"=w361:string)  [unwired: 7 in]
        n135 = call <vilib>:"Add State(s) to Queue__jki_lib_state_machine.vi"("State(s) in (\"\")"=w361, "State(s) at Back (\"\")"="UI: Uninitialize\nData: Cleanup\nEvents: Unregister\nExit") -> ("States Out"=w365:string)  [unwired: 13 in]
        n136 = call <vilib>:"Add State(s) to Queue__jki_lib_state_machine.vi"("State(s) in Front (\"\")"=w365, "State(s) in (\"\")"=w369) -> ("States Out"=w368:string)  [unwired: 13 in]
      }
      frame "---------- Action ----------" {
        n137 = call <vilib>:"Add State(s) to Queue__jki_lib_state_machine.vi"("State(s) in (\"\")"=w374) -> ("States Out"=w373:string)  [unwired: 14 in]
      }
      frame "Action: Queue Publisher" {
        n138 = Unbundle By Name(w391) -> ("job queue"=w379:refnum<queue>, "manager_daemon"=w384:refnum<class "manager_daemon.lvclass">, "cv_pub path"=w386:path)
        n139 = Format Into String(format string="%d.json", "Publisher ID") -> (resulting string=w389:string)  [unwired: 2 in, 1 out]
        n140 = Build Path(base path=w386, name or relative path=w389) -> (appended path=w388:path)
        n141 = call "open.local.publisher.file.vi"("error in (no error)"=w385, "publisher json"=w388) -> ("error out"=w383:errorcluster, "publisher"=w387:T7)  [unwired: 8 in]
        n142 = Unbundle By Name(w387) -> ("volume_ids"=w381:i32[])
        n143 = call "get volume ids by publisher.vi"("error in (no error)"=w383, "publisher id"="Publisher ID", "manager_daemon in"=w384) -> ("error out"=w378:errorcluster, "volume ids"=w380:i32[])  [unwired: 6 in, 1 out]
        n144 = for {
          tunnel: w381 -> [w395] mode=indexing
          tunnel: w380 -> [w402]
          tunnel: w379 -> [w400]
          shift-right: [w398] -> w375
          shift-left: w378 -> [w399]
          tunnel: T2 {"job type"=enum."check volume date", "job path"=path "", "id"=0, "url"="", "last updated"=timestamp(0 s since 1904-01-01), "offset"=0, "original path"=path ""} ("element") -> [w397]
          tunnel: job_type--enum."download volume" ("job type") -> [w396]
          n145 = Search 1D Array(1D array=w402, element=w395) -> (index of element=w401:i32)  [unwired: 1 in]
          n146 = case shown="Default" w401 {
            tunnel: w400 -> [_ w410]
            tunnel: w399 -> [w403 w409]
            tunnel: [w403 w408] -> w398
            tunnel: w397 -> [_ w407]
            tunnel: w396 -> [_ w406]
            tunnel: w395 -> [_ w405]
            frame Default {
            }
            frame -1 {
              n147 = Bundle By Name(cluster=w407, "job type"=w406, "id"=w405) -> (w404:T2)
              n148 = Enqueue Element(queue=w410, element=w404, error in (no error)=w409) -> (error out=w408:errorcluster)  [unwired: 1 in, 2 out]
            }
          }
        }
        n149 = call <vilib>:"Add State(s) to Queue__jki_lib_state_machine.vi"("State(s) in (\"\")"=w394) -> ("States Out"=w393:string)  [unwired: 14 in]
      }
      frame "Action: Reset dl timer" {
        n150 = Unbundle By Name(w431) -> ("ms delay"=w419:u32, "crawler active"=w428:bool, "job queue"=w430:refnum<queue>, "cache folder"=w415:path)
        n151 = Tick Count (ms)() -> (millisecond timer value=w433:u32)
        n152 = Add(x=w433, y=w419) -> (x+y=w432:u32)
        n153 = call "get_next_job.vi"("error in (no error)"=w416, "cache path"=w415) -> ("error out"=w417:errorcluster, "remaining jobs"=w414:i32)  [unwired: 7 in, 1 out]
        n154 = Bundle By Name(cluster=w431, "dl timer"=w432) -> (w420:T5)
        n155 = Equal To 0?(x=w414) -> (x = 0?=w413:bool)
        n156 = Get Queue Status(queue=w430, error in (no error)=w417) -> (error out=w422:errorcluster, # elements in queue=w429:i32)  [unwired: 1 in, 6 out]
        n157 = Equal To 0?(x=w429) -> (x = 0?=w425:bool)
        n158 = call "init_logs.vi"("error in (no error)"=w422, "Cluster in"=w420) -> ("error out"=w421:errorcluster, "Cluster out"=w423:T5)  [unwired: 8 in]
        n159 = Compound Arithmetic op=AND(w425, w413) -> (w426:bool)
        n160 = case shown="True" w426 {
          tunnel: w428 -> [w441 _]
          tunnel: w425 -> [w440 _]
          tunnel: [w439 _] -> w427
          tunnel: w423 -> [w438 w455]
          tunnel: [w438 w454] -> w424
          tunnel: "pause" -> [w437 _]
          tunnel: [w436 "Reset timer: Inactive" ("status")] -> w411
          frame False {
            n161 = case shown="True" w437 {
              tunnel: w441 -> [w447 _]
              tunnel: w440 -> [w445 _]
              tunnel: [w443 _] -> w439
              tunnel: ["Action: Reset dl timer" ("status") "Downloading Paused" ("status")] -> w436
              frame False {
                n162 = And(x=w447, y=w445) -> (x .and. y?=w446:bool)
                n163 = call <vilib>:"Conditional State String__jki_lib_state_machine.vi"("Do State(s)?"=w446, "State"="Action: Process Next Batch\nAction: Run Job") -> ("State Out"=w444:string)  [unwired: 7 in]
                n164 = case shown="False" w445 {
                  tunnel: w444 -> [_ w450]
                  tunnel: ["Action: Run Job" ("State Out") w450] -> w443
                  frame False {
                  }
                  frame True {
                  }
                }
              }
              frame True {
              }
            }
          }
          frame True {
            n165 = Bundle By Name(cluster=w455, "crawler active"=FALSE) -> (w454:T5)
          }
        }
        n166 = local write "status"(w411) -> ()
        n167 = call <vilib>:"Add State(s) to Queue__jki_lib_state_machine.vi"("State(s) in Front (\"\")"=w427, "State(s) in (\"\")"=w435) -> ("States Out"=w434:string)  [unwired: 13 in]
      }
      frame "Action: Process Next Batch" {
        n168 = Unbundle By Name(w457) -> ("cache folder"=w461:path, "job queue"=w459:refnum<queue>)  [unwired: 1 out]
        n169 = call "create_vol_and_issue_date_job.vi"("error in (no error)"=w460, "job queue"=w459, "job path"=w461) -> ("error out"=w458:errorcluster)  [unwired: 6 in, 2 out]
        n170 = local write "status"("Action: Process Next Batch" ("status")) -> ()
        n171 = call <vilib>:"Add State(s) to Queue__jki_lib_state_machine.vi"("State(s) in (\"\")"=w464) -> ("States Out"=w463:string)  [unwired: 14 in]
      }
      frame "Action: Add Volume Manually" {
        n172 = Unbundle By Name(w474) -> ("cv_pub path"=w465:path, "job queue"=w477:refnum<queue>, "manager_daemon"=w472:refnum<class "manager_daemon.lvclass">, "cv_iss path"=w473:path)
        n173 = call <vilib>:"Trim Whitespace.vi"("string"="Volume URL") -> ("trimmed string"=w466:string)  [unwired: 1 in]
        n174 = call <userlib>:"String to 1D Array__ogtk.vi"("delimiter (Tab)"="\n", "string"=w466) -> ("Array of Strings"=w468:string[])  [unwired: 9 in]
        n175 = Reverse 1D Array(array=w468) -> (reversed array=w467:string[])
        n176 = for {
          tunnel: w478 -> [w489]
          tunnel: w477 -> [w488]
          tunnel: [w487] -> w476
          tunnel: [w486] -> w475
          tunnel: w473 -> [w485]
          tunnel: w472 -> [w484]
          tunnel: w467 -> [w483] mode=indexing
          tunnel: w465 -> [w482]
          n177 = call "add_url_manually.vi"("Volume URL in"=w483, "cv_pub path"=w482, "error in (no error)"=w489, "cv_issue path"=w485, "manager_daemon"=w484, "Queue in"=w488) -> ("error out"=w487:errorcluster, "Volume URL out"=w486:string)  [unwired: 4 in]
        }
        n178 = local write "status"("Action: Add Volume Manually" ("status")) -> ()
        n179 = local write "Volume URL"(w475) -> ()
        n180 = call <vilib>:"Add State(s) to Queue__jki_lib_state_machine.vi"("State(s) in (\"\")"=w481) -> ("States Out"=w480:string)  [unwired: 14 in]
      }
      frame "Action: Stop Crawler" {
        n181 = Unbundle By Name(w492) -> ("job queue"=w496:refnum<queue>)
        n182 = Flush Queue(queue=w496, error in (no error)=w495) -> (error out=w494:errorcluster)  [unwired: 2 out]
        n183 = local write "status"("Action: Stop Crawler" ("status")) -> ()
        n184 = Bundle By Name(cluster=w492, "crawler active"=FALSE) -> (w493:T5)
        n185 = call <vilib>:"Add State(s) to Queue__jki_lib_state_machine.vi"("State(s) in (\"\")"=w499) -> ("States Out"=w498:string)  [unwired: 14 in]
      }
      frame "Action: Run Job" {
        n186 = Unbundle By Name(w528) -> ("cv_vol path"=w501:path, "cv_pub path"=w500:path, "cv_iss path"=w524:path, "REST Client"=w529:refnum<class "REST Client.lvclass">, "job queue"=w503:refnum<queue>, "manager_daemon"=w525:refnum<class "manager_daemon.lvclass">, "status log ref"=w515:refnum<file>, "ms delay"=w504:u32)
        n187 = local read "files updated"() -> (w522:string[])
        n188 = Divide(x=w504, y=1000.0) -> (x/y=w510:dbl)
        n189 = call "run_job.vi"("REST Client in"=w529, "issue folder path"=w524, "pub folder path"=w500, "volume folder path"=w501, "job queue"=w503, "manager_daemon"=w525, "error in (no error)"=w530, "files updated"=w522) -> ("REST Client out"=w526:refnum<class "REST Client.lvclass">, "Run Next"=w520:bool, "status"=w512:string, "job path"=w513:path, "files updated out"=→"files updated":string[], "error out"=w523:errorcluster)  [unwired: 1 in, 1 out]
        n190 = Get Queue Status(queue=w503) -> (# elements in queue=w502:i32)  [unwired: 2 in, 7 out]
        n191 = call "clear_job.vi"("last job"=w513, "error in (no error)"=w523) -> ("error out"=w517:errorcluster)  [unwired: 9 in]
        n192 = Get Date/Time In Seconds() -> (seconds since 1Jan1904=w509:timestamp)
        n193 = Multiply(x=w502, y=w510) -> (x*y=w507:dbl)
        n194 = Greater Than 0?(x=w502) -> (x > 0?=w506:bool)
        n195 = call "Write String to Log.vi"("error in (no error)"=w517, "Information"=w512, "file reference in"=w515) -> ("error out"=w516:errorcluster, "file reference out"=w514:refnum<file>)  [unwired: 7 in]
        n196 = local write "status"(w512) -> ()
        n197 = Add(x=w507, y=w509) -> (x+y=→"Approx Completion":timestamp)
        n198 = Bundle By Name(cluster=w528, "REST Client"=w526, "status log ref"=w514) -> (w527:T5)
        n199 = property on="Approx Completion" class="AbsTime (strict)"("Visible"=w506) -> ()  [unwired: 2 in, 2 out]
        n200 = call <vilib>:"Conditional State String__jki_lib_state_machine.vi"("Do State(s)?"=w520, "State"="Action: Run Job") -> ("State Out"=w518:string)  [unwired: 7 in]
        n201 = call <vilib>:"Add State(s) to Queue__jki_lib_state_machine.vi"("State(s) in Front (\"\")"=w518, "State(s) in (\"\")"=w532) -> ("States Out"=w531:string)  [unwired: 13 in]
      }
      frame "Action: Populate Log Folder" {
        n202 = Unbundle By Name(w537) -> ("cv_vol path"=w540:path, "cache folder"=w545:path)
        n203 = Build Path(base path=w545, name or relative path=path "jobs") -> (appended path=w544:path)
        n204 = case shown="False" "Rebuild Job List" {
          tunnel: w544 -> [w550 w554]
          tunnel: w543 -> [w549 w553]
          tunnel: [w549 w552] -> w542
          tunnel: [w550 w551] -> w541
          frame False {
          }
          frame True {
            n205 = call "ClearWorkingDirectory.vi"("error in"=w553, "Working Path"=w554) -> ("error out"=w552:errorcluster, "Working Path Out"=w551:path)  [unwired: 8 in]
          }
        }
        n206 = local write "status"("Action: Populate Log Folder" ("status")) -> ()
        n207 = call "populate_volume_cache.vi"("rebuild job list"="Rebuild Job List", "error in (no error)"=w542, "job path"=w541, "cv_vol path"=w540) -> ("error out"=w539:errorcluster)  [unwired: 7 in]
        n208 = Bundle By Name(cluster=w537, "crawler active"=TRUE) -> (w536:T5)
        n209 = call <vilib>:"Add State(s) to Queue__jki_lib_state_machine.vi"("State(s) in (\"\")"=w548) -> ("States Out"=w547:string)  [unwired: 14 in]
      }
    }
  }
